vi "Upstream Error Message.vi"() -> (3 "Upstream Error Message":string="An error occurred upstream.")   [LabVIEW 2017, in "Git-LabVIEW.lvlib" / "Git Implementation.lvclass"]
doc: "Provide a message for the Error case in API operations, when the operation receives an error on the input wire."
uses:
  Git Implementation.lvclass
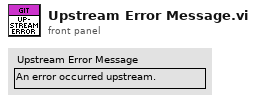
[diagram p1: front panel]
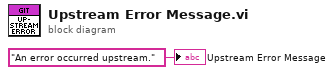
[diagram p0: block diagram]
diagram:
  "Upstream Error Message" <- "An error occurred upstream." ("StdOut")
